vi "Check for Start Position.vi"(7 "Cancel Inspect":bool, 8 "error in (no error)":errorcluster, 9 "Target Encdr Pos.":i32, 10 "Cur Encoder Value":i32, 11 "Status Byte":u16) -> (0 "error out":errorcluster, 1 "Aborted":bool, 2 "Cancelled":bool, 3 "Success":bool, 4 "Log String out":string)   [LabVIEW 2015, in "Tool Module.lvlib"]
uses:
  Tool Module.lvlib
  <vilib>/Utility/error.llb/Error Cluster From Error Code.vi
  <vilib>/ErrorRing/Error Ring.xnode
  Tool Interface/Tool Interface.lvlib
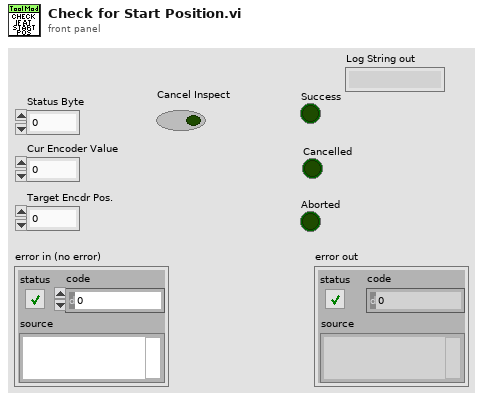
[diagram p1: front panel]
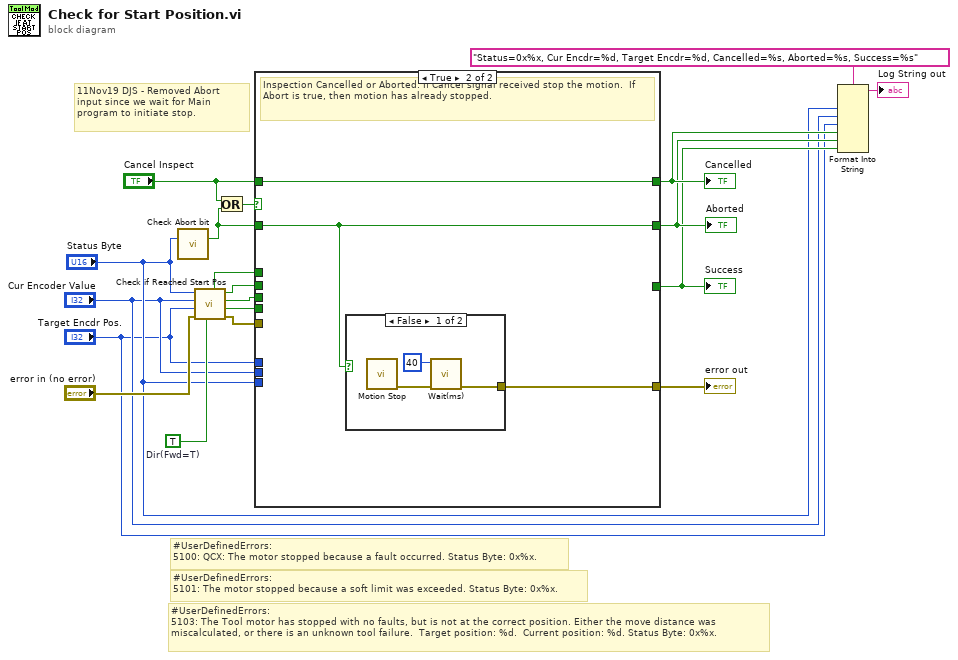
[diagram p0: block diagram]
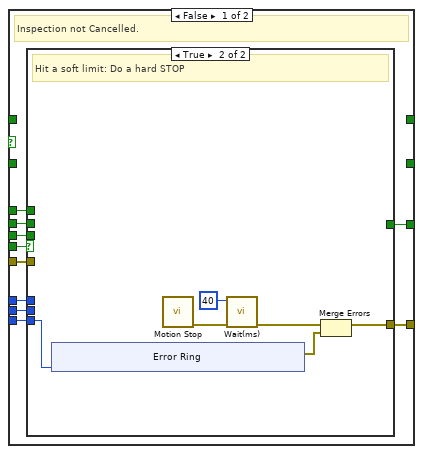
[diagram p2: hidden frame]
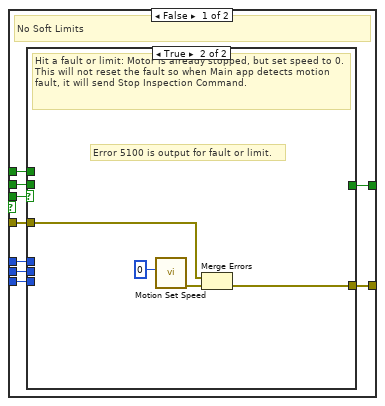
[diagram p3: hidden frame]
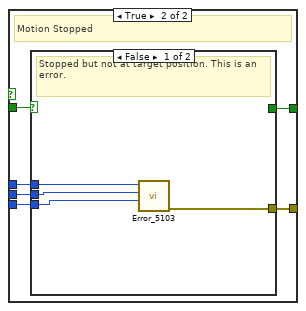
[diagram p5: hidden frame]
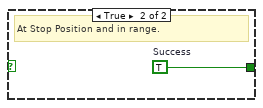
[diagram p6: hidden frame]
diagram:
  w12 = TRUE  # Dir(Fwd=T)
  # "11Nov19 DJS - Removed Abort input since we wait for Main program to initiate stop."
  # "#UserDefinedErrors:\n5101: The motor stopped because a soft limit was exceeded. Status Byte: 0x%x."
  # "#UserDefinedErrors:\n5100: QCX: The motor stopped because a fault occurred. Status Byte: 0x%x."
  # "#UserDefinedErrors:\n5103: The Tool motor has stopped with no faults, but is not at the correct position. Either the move distance was miscalculated, or there is an unknown tool failure.  Target position: %d.  Current position: %d. Status Byte: 0x%x."
  n1 = call "Check Abort bit.vi"("Status Byte"="Status Byte") -> ("Abort?"=w1:bool)  [unwired: 14 in]
  n2 = call "Check if Reached Start Pos.vi"("Dir(Fwd=T)"=w12, "error in (no error)"="error in (no error)", "Target Encdr Pos."="Target Encdr Pos.", "Cur Encoder Value"="Cur Encoder Value", "Status Byte"="Status Byte") -> ("error out"=w15:errorcluster, "Soft Limit?"=w19:bool, "Fault or Hard Limit"=w18:bool, "ReachedPos?"=w17:bool, "MotionStopped?"=w16:bool)  [unwired: 2 in]
  n3 = Or(x="Cancel Inspect", y=w1) -> (x .or. y?=w11:bool)
  n4 = case shown="True" w11 {
    tunnel: w19 -> [w29 _]
    tunnel: w18 -> [w28 _]
    tunnel: w17 -> [w27 _]
    tunnel: [_ w74] -> w9
    tunnel: [w26 _] -> w7
    tunnel: w16 -> [w25 _]
    tunnel: [w24 w76] -> w14
    tunnel: "Target Encdr Pos." -> [w23 _]
    tunnel: "Cur Encoder Value" -> [w22 _]
    tunnel: "Status Byte" -> [w21 _]
    tunnel: w15 -> [w20 _]
    tunnel: w1 -> [_ w75]
    tunnel: [_ w75] -> w8
    tunnel: "Cancel Inspect" -> [_ w74]
    frame False {
      # "Inspection not Cancelled."
      n5 = case shown="True" w29 {
        tunnel: w28 -> [w38 _]
        tunnel: w27 -> [w37 _]
        tunnel: [w36 _] -> w26
        tunnel: w25 -> [w35 _]
        tunnel: [w34 w63] -> w24
        tunnel: w23 -> [w33 _]
        tunnel: w22 -> [w32 _]
        tunnel: w21 -> [w31 w61]
        tunnel: w20 -> [w30 _]
        frame False {
          # "No Soft Limits"
          n6 = case shown="True" w38 {
            tunnel: w37 -> [w43 _]
            tunnel: [w45 _] -> w36
            tunnel: w35 -> [w44 _]
            tunnel: [w42 w58] -> w34
            tunnel: w33 -> [w41 _]
            tunnel: w32 -> [w40 _]
            tunnel: w31 -> [w39 _]
            tunnel: w30 -> [_ w57]
            frame False {
              # "No Fault"
              n7 = case shown="False" w44 {
                tunnel: [_ w50] -> w45
                tunnel: w43 -> [_ w51]
                tunnel: [_ w49] -> w42
                tunnel: w41 -> [_ w48]
                tunnel: w40 -> [_ w47]
                tunnel: w39 -> [_ w46]
                frame False {
                  # "Still moving -- loop again."
                }
                frame True {
                  # "Motion Stopped"
                  n8 = case shown="False" w51 {
                    tunnel: [_ w56] -> w50
                    tunnel: [w55 _] -> w49
                    tunnel: w48 -> [w54 _]
                    tunnel: w47 -> [w53 _]
                    tunnel: w46 -> [w52 _]
                    frame False {
                      # "Stopped but not at target position. This is an error."
                      n9 = call "Error_5103.vi"("Status"=w52, "Current Pos"=w53, "Target Pos"=w54) -> ("error out"=w55:errorcluster)  [unwired: 8 in]
                    }
                    frame True {
                      w56 = TRUE  # Success
                      # "At Stop Position and in range."
                    }
                  }
                }
              }
            }
            frame True {
              # "Error 5100 is output for fault or limit."
              # "Hit a fault or limit: Motor is already stopped, but set speed to 0. This will not reset the fault so when Main app detects motion fault, it will send Stop Inspection Command."
              n10 = call "Motion Set Speed.vi"("Speed"=u16 0) -> ("error out"=w59:errorcluster)  [unwired: 10 in]
              n11 = Merge Errors(w57, w59) -> (w58:errorcluster)
            }
          }
        }
        frame True {
          # "Hit a soft limit: Do a hard STOP"
          n12 = xnode "Error Ring"("parameter 0"=w61) -> ("error out"=w62:errorcluster)
          n13 = call "Motion Stop.vi"() -> ("error out"=w66:errorcluster)  [unwired: 11 in]
          n14 = call "Wait(ms).vi"("error in (no error)"=w66, "milliseconds"=u32 40) -> ("error out"=w64:errorcluster)  [unwired: 9 in]
          n15 = Merge Errors(w64, w62) -> (w63:errorcluster)
        }
      }
    }
    frame True {
      # "Inspection Cancelled or Aborted. If Cancel signal received stop the motion.  If Abort is true, then motion has already stopped."
      n16 = case shown="False" w75 {
        tunnel: [w77 _] -> w76
        frame False {
          n17 = call "Motion Stop.vi"() -> ("error out"=w79:errorcluster)  [unwired: 11 in]
          n18 = call "Wait(ms).vi"("error in (no error)"=w79, "milliseconds"=u32 40) -> ("error out"=w77:errorcluster)  [unwired: 9 in]
        }
        frame True {
        }
      }
    }
  }
  "Cancelled" <- w9
  "Success" <- w7
  "error out" <- w14
  "Aborted" <- w8
  n19 = Format Into String(format string="Status=0x%x, Cur Encdr=%d, Target Encdr=%d, Cancelled=%s, Aborted=%s, Success=%s", "Status Byte", "Cur Encoder Value", "Target Encdr Pos.", w9, w8, w7) -> (resulting string=→"Log String out":string)  [unwired: 2 in, 1 out]
